vi "GdsLanguage_LoadLanguages.vi"(0 "LanguageFilesDirectory":path, 2 "LanguagesToLoad":T2, 3 "ChesumControl":T1, 5 "error in (no error)":errorcluster) -> (13 "StringIDsMissingThisLangaugeTranslation":string[](array[string]), 14 "StringIDArray":string[](array[string]), 16 "TranslatedStrings":string[](array[string]), 17 "DuplicateTranslations":string[](array[string]), 18 "FoundLanguages":T2[](array[typedef]), 19 "error out":errorcluster)   [LabVIEW 2020]
doc: "Load the languages (translated strings)."
uses:
  <resource>/Framework/Providers/Open_GDS/ClassProviders/Common/GdsLanguage/GdsLanguage_LanguageID.ctl
  <resource>/Framework/Providers/Open_GDS/ClassProviders/Common/GdsLanguage/private/GdsLanguage_ChecksumCheckType.ctl
  <resource>/Framework/Providers/Open_GDS/SubVIs/GOOP_ErrorCodes.ctl
  <vilib>/Utility/config.llb/Read Key (String).vi
  <vilib>/Utility/config.llb/NI_LVConfig.lvlib
panel:
  out "descriptions":string[](array[string])
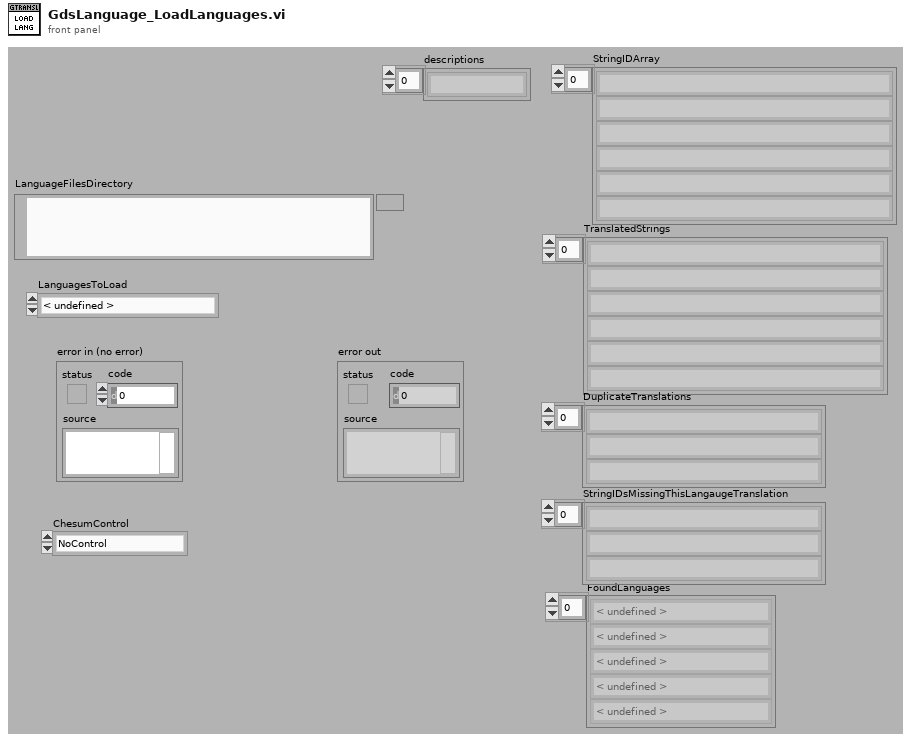
[diagram p1: front panel]
types:
  T1 = typedef "GdsLanguage_ChecksumCheckType.ctl" = enum16{"NoControl", "CheckChecksum", "AddChecksum"}
  T2 = typedef "GdsLanguage_LanguageID.ctl" = enum16{"< undefined >", "aa", "ab", "af", "am", "ar", "as", "ay", "az", "ba", "be", "bg", "bh", "bi", "bn", "bo", "br", "ca", "co", "cs", "cy", "da", "de", "dz", "el", "en", "eo", "es", "et", "eu", "fa", "fi", "fj", "fo", "fr", "fy", "ga", "gd", "gl", "gn", "gu", "gv", "ha", "he", "hi", "hr", "hu", "hy", "ia", "id", "ie", "ik", "is", "it", "iu", "ja", "jv", "ka", "kk", "kl", "km", "kn", "ko", "ks", "ku", "ky", "la", "li", "ln", "lo", "lt", "lv", "mg", "mi", "mk", "ml", "mn", "mo", "mr", "ms", "mt", "my", "na", "ne", "nl", "no", "oc", "om", "or", "pa", "pl", "ps", "pt", "qu", "rm", "rn", "ro", "ru", "rw", "sa", "sd", "sg", "sh", "si", "sk", "sl", "sm", "sn", "so", "sq", "sr", "ss", "st", "su", "sv", "sw", "ta", "te", "tg", "th", "ti", "tk", "tl", "tn", "to", "tr", "ts", "tt", "tw", "ug", "uk", "ur", "uz", "vi", "vo", "wo", "xh", "yi", "yo", "zh", "zu"}
  T3 = typedef "GOOP_ErrorCodes.ctl" = enum16{"LicenseFileMissing", "LicenseFileNotCorrect", "NoProductAccessGranted", "AgreementNoAccepted", "NoValidProviderFound", "LicenseExpired", "LanguageUndefined", "LanguageFileMissing", "LanguageFileChecksumError", "DublicateLanguageTranslation", "LanguageStringIDNotFound", "CommunityLimitReached", "ClassFileLocked", "ClassFileReadOnly", "ProjectNotValid"}
  T4 = typedef "NI_LVConfig.lvlib/Config Data RefNum.ctl" = refnum<k1>
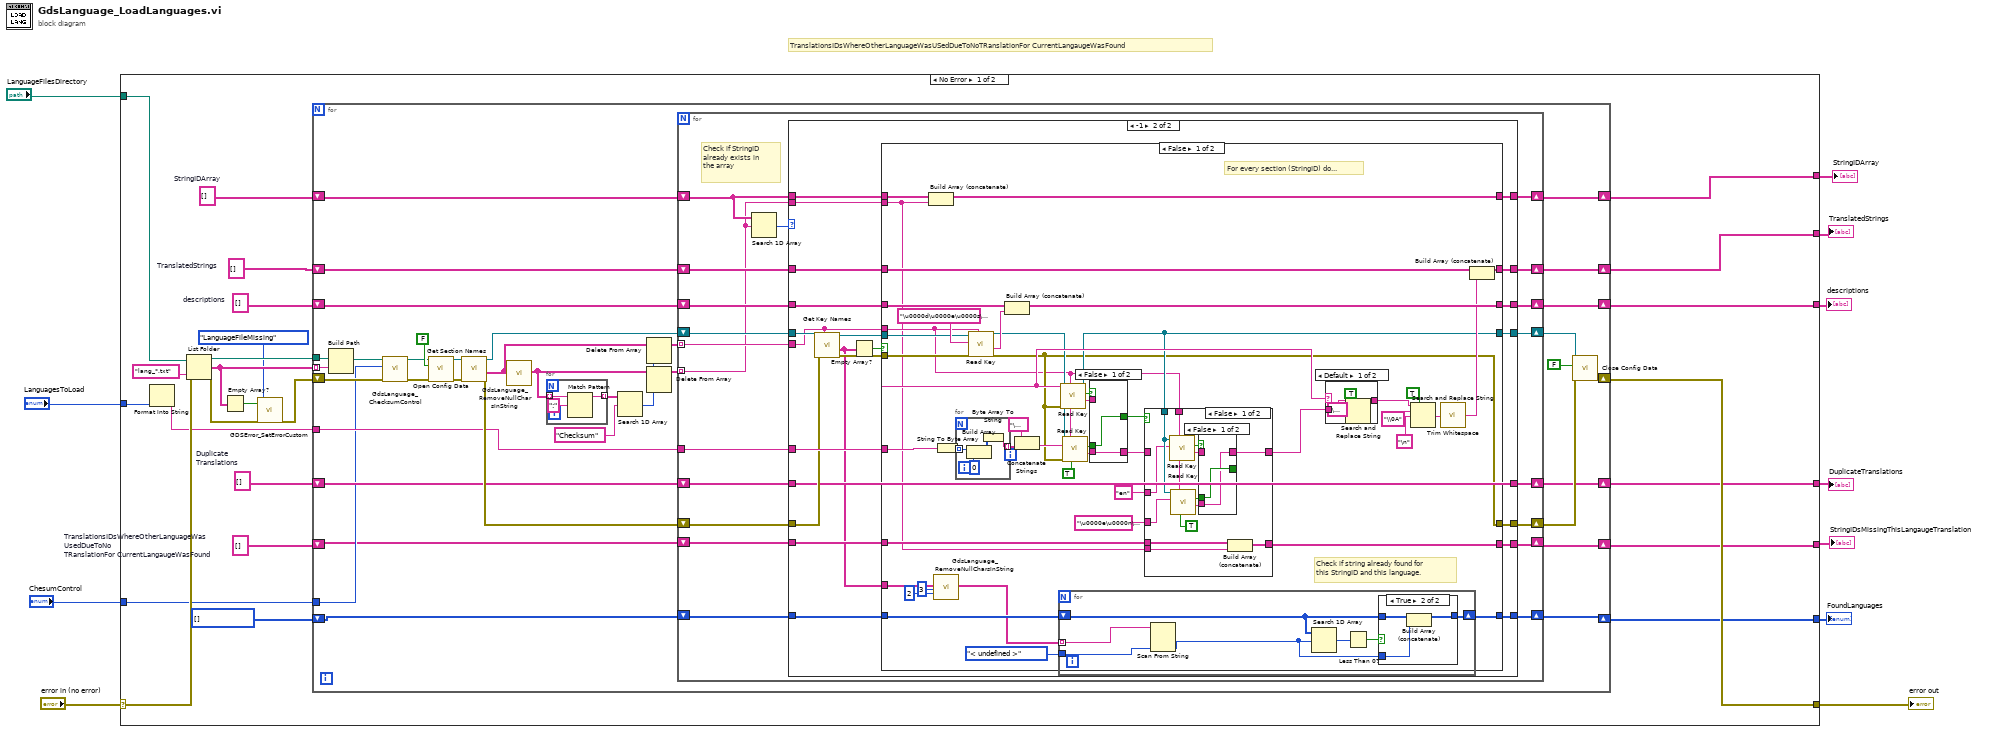
[diagram p0: block diagram]
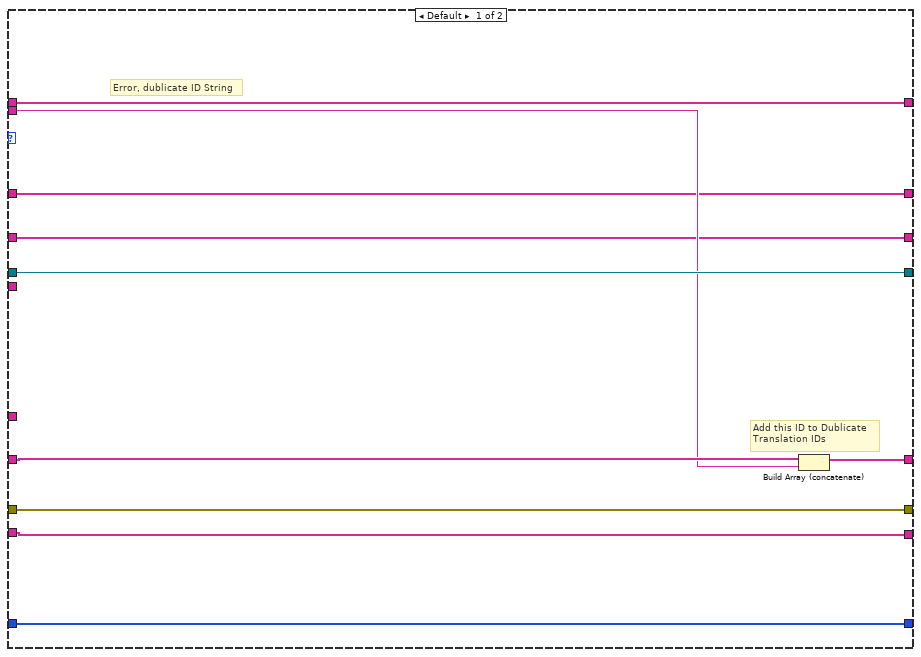
[diagram p2: hidden frame]
diagram:
  # "TranslationsIDsWhereOtherLanguageWasUSedDueToNoTRanslationFor CurrentLangaugeWasFound"
  n1 = case shown="No Error" "error in (no error)" {
    selector: "error in (no error)" -> [w32 w223]
    tunnel: [w33 w223] -> w10
    tunnel: "LanguageFilesDirectory" -> [w35 _]
    tunnel: "LanguagesToLoad" -> [w20 _]
    tunnel: [w29 _] -> w2
    tunnel: [w28 _] -> w7
    tunnel: [w26 _] -> w6
    tunnel: [w22 _] -> w5
    tunnel: [w23 _] -> w4
    tunnel: "ChesumControl" -> [w21 _]
    tunnel: [w17 _] -> w1
    frame No Error {
      w18 = string[] []  # TranslationsIDsWhereOtherLanguageWas UsedDueToNo TRanslationFor CurrentLangaugeWasFound
      w24 = string[] []  # descriptions
      w25 = T2[] [] items=["< undefined >", "aa", "ab", "af", "am", "ar", "as", "ay", "az", "ba", "be", "bg", "bh", "bi", "bn", "bo", "br", "ca", "co", "cs", "cy", "da", "de", "dz", "el", "en", "eo", "es", "et", "eu", "fa", "fi", "fj", "fo", "fr", "fy", "ga", "gd", "gl", "gn", "gu", "gv", "ha", "he", "hi", "hr", "hu", "hy", "ia", "id", "ie", "ik", "is", "it", "iu", "ja", "jv", "ka", "kk", "kl", "km", "kn", "ko", "ks", "ku", "ky", "la", "li", "ln", "lo", "lt", "lv", "mg", "mi", "mk", "ml", "mn", "mo", "mr", "ms", "mt", "my", "na", "ne", "nl", "no", "oc", "om", "or", "pa", "pl", "ps", "pt", "qu", "rm", "rn", "ro", "ru", "rw", "sa", "sd", "sg", "sh", "si", "sk", "sl", "sm", "sn", "so", "sq", "sr", "ss", "st", "su", "sv", "sw", "ta", "te", "tg", "th", "ti", "tk", "tl", "tn", "to", "tr", "ts", "tt", "tw", "ug", "uk", "ur", "uz", "vi", "vo", "wo", "xh", "yi", "yo", "zh", "zu"] ("Array out (String)")
      w27 = string[] []  # Duplicate Translations
      w30 = string[] []  # TranslatedStrings
      w31 = string[] []  # StringIDArray
      n2 = Format Into String(w20) -> (resulting string=w19:string)  [unwired: 3 in, 1 out]
      n3 = List Folder(path=w35, pattern="lang_*.txt", error in=w32) -> (path out=w34:path, filenames=w16:string[], error out=w13:errorcluster)  [unwired: 1 in, 1 out]
      n4 = Empty Array?(array=w16) -> (empty?=w14:bool)
      n5 = call <resource>:"GDSError_SetErrorCustom.vi"("status"=w14, "error in (no error)"=w13, "UserDefinedCodes(+5000)"=GOOP_ErrorCodes."LanguageFileMissing") -> ("error out"=w12:errorcluster)  [unwired: 16 in]
      n6 = for {
        tunnel: w34 -> [w65]
        tunnel: w16 -> [w64] mode=indexing
        tunnel: w19 -> [w63]
        shift-right: [w62] -> w33
        shift-left: w12 -> [w49]
        shift-right: [w59] -> w28
        shift-left: w31 -> [w61]
        shift-right: [w58] -> w29
        shift-left: w30 -> [w60]
        shift-right: [w56] -> w26
        shift-left: w27 -> [w57]
        shift-right: [w54] -> w22
        shift-left: w25 -> [w53]
        shift-right: [w51] -> w23
        shift-left: w24 -> [w52]
        tunnel: w21 -> [w46]
        shift-right: [w45] -> w17
        shift-left: w18 -> [w44]
        n7 = Build Path(base path=w65, name or relative path=w64) -> (appended path=w50:path)
        n8 = call <resource>:"GdsLanguage_ChecksumControl.vi"("error in"=w49, "ChesumControl"=w46, "LanguangeFileIn"=w50) -> ("error out"=w47:errorcluster, "LanguangeFileOut"=w48:path)  [unwired: 7 in]
        n9 = call <vilib>:"Open Config Data.vi"("error in (no error)"=w47, "create file if necessary (T)"=FALSE ("create file if necessary? (T)"), "configuration file path"=w48) -> ("error out"=w68:errorcluster, "refnum"=w72:T4)  [unwired: 6 in, 1 out]
        n10 = call <vilib>:"Get Section Names.vi"("error in (no error)"=w68, "refnum"=w72) -> ("error out"=w67:errorcluster, "section names"=w41:string[], "refnum out"=w70:T4)  [unwired: 7 in]
        n11 = call <resource>:"GdsLanguage_RemoveNullCharsInString.vi"("StringArray-IN"=w41) -> ("StringArray-Out"=w39:string[])  [unwired: 18 in]
        n12 = for {
          tunnel: w39 -> [w75] mode=indexing
          tunnel: [w73] -> w43 mode=indexing
          n13 = Match Pattern(string=w75, regular expression=":") -> (before substring=w73:string)  [unwired: 1 in, 3 out]
        }
        n14 = Search 1D Array(1D array=w43, element="Checksum") -> (index of element=w37:i32)  [unwired: 1 in]
        n15 = Delete From Array(array=w41, index=w37) -> (array with subset deleted=w40:string[])  [unwired: 1 in, 1 out]
        n16 = Delete From Array(array=w39, index=w37) -> (array with subset deleted=w38:string[])  [unwired: 1 in, 1 out]
        n17 = for {
          tunnel: w38 -> [w79] mode=indexing
          shift-right: [w95] -> w69
          shift-left: w70 -> [w87]
          tunnel: w63 -> [w94]
          shift-right: [w93] -> w66
          shift-left: w67 -> [w88]
          shift-right: [w78] -> w59
          shift-left: w61 -> [w80]
          shift-right: [w91] -> w58
          shift-left: w60 -> [w92]
          shift-right: [w89] -> w56
          shift-left: w57 -> [w90]
          shift-right: [w83] -> w54
          shift-left: w53 -> [w82]
          shift-right: [w85] -> w51
          shift-left: w52 -> [w86]
          tunnel: w40 -> [w84] mode=indexing
          shift-right: [w77] -> w45
          shift-left: w44 -> [w76]
          # "Check if StringID already exists in the array"
          n18 = Search 1D Array(1D array=w80, element=w79) -> (index of element=w81:i32)  [unwired: 1 in]
          n19 = case shown="-1" w81 {
            tunnel: [w102 w109] -> w95
            tunnel: w94 -> [_ w127]
            tunnel: [w103 w108] -> w93
            tunnel: w92 -> [w97 w126]
            tunnel: [w97 w125] -> w91
            tunnel: w90 -> [w104 w114]
            tunnel: [w105 w114] -> w89
            tunnel: w88 -> [w103 w124]
            tunnel: w87 -> [w102 w123]
            tunnel: w86 -> [w98 w122]
            tunnel: [w98 w119] -> w85
            tunnel: w84 -> [_ w110]
            tunnel: [w99 w118] -> w83
            tunnel: w82 -> [w99 w117]
            tunnel: w80 -> [w100 w116]
            tunnel: w79 -> [w101 w115]
            tunnel: [w100 w113] -> w78
            tunnel: [w96 w112] -> w77
            tunnel: w76 -> [w96 w111]
            frame Default {
              # "Add this ID to Dublicate\nTranslation IDs"
              # "Error, dublicate ID String"
              n20 = Build Array (concatenate)(w104, w101) -> (w105:string[])
            }
            frame -1 {
              n21 = call <vilib>:"Get Key Names.vi"("section"=w110, "error in (no error)"=w124, "refnum"=w123) -> ("error out"=w120:errorcluster, "key names"=w107:string[], "refnum out"=w121:T4)  [unwired: 5 in, 1 out]
              n22 = Empty Array?(array=w107) -> (empty?=w106:bool)
              n23 = case shown="False" w106 {
                tunnel: w127 -> [w172 _]
                tunnel: w126 -> [w171 w221]
                tunnel: [w170 w221] -> w125
                tunnel: w122 -> [w167 w220]
                tunnel: w121 -> [w166 w219]
                tunnel: w120 -> [w164 w218]
                tunnel: [w163 w220] -> w119
                tunnel: [w160 w216] -> w118
                tunnel: w117 -> [w159 w216]
                tunnel: w116 -> [w148 w222]
                tunnel: w115 -> [w130 _]
                tunnel: [w147 w222] -> w113
                tunnel: [w139 w217] -> w112
                tunnel: w111 -> [w138 w217]
                tunnel: w110 -> [w131 _]
                tunnel: [w137 w219] -> w109
                tunnel: [w134 w218] -> w108
                tunnel: w107 -> [w133 _]
                frame False {
                  # "Check if string already found for \nthis StringID and this language."
                  # "For every section (StringID) do..."
                  n24 = Build Array (concatenate)(w148, w130) -> (w147:string[])
                  n25 = call <resource>:"GdsLanguage_RemoveNullCharsInString.vi"("StringArray-IN"=w133, "MaxLengthLimit(ignored if not wired)"=3, "MinLengthLimit(ignored if not wired)"=2) -> ("StringArray-Out"=w132:string[])  [unwired: 16 in]
                  n26 = String To Byte Array(string=w172) -> (unsigned byte array=w151:u8[])
                  n27 = for {
                    tunnel: w151 -> [w204] mode=indexing
                    tunnel: [w202] -> w157 mode=indexing
                    n28 = Build Array(w204, u8 0 ("element")) -> (w203:u8[])
                    n29 = Byte Array To String(unsigned byte array=w203) -> (string=w202:string)
                  }
                  n30 = call-poly <vilib>:"Read Key.vi"("section"=w131, "error in (no error)"=w164, "key"="\u0000d\u0000e\u0000s\u0000c\u0000r\u0000i\u0000p\u0000t\u0000i\u0000o\u0000n\u0000", "refnum"=w166) -> ("error out"=w134:errorcluster, "value"=w168:string, "refnum out"=w165:T4)  [unwired: 4 in, 1 out]
                  n31 = Build Array (concatenate)(w167, w168) -> (w163:string[])
                  n32 = Concatenate Strings("\u0000" ("string"), w157) -> (w154:string)
                  n33 = for {
                    shift-right: [w209] -> w160
                    shift-left: w159 -> [w210]
                    tunnel: w132 -> [w207] mode=indexing
                    tunnel: GdsLanguage_LanguageID."< undefined >" ("LanguagesToLoad") -> [w206]
                    n34 = Scan From String(input string=w207, default 1=w206) -> (output 1=w205:T2)  [unwired: 3 in, 3 out]
                    n35 = Search 1D Array(1D array=w210, element=w205) -> (index of element=w208:i32)  [unwired: 1 in]
                    n36 = Less Than 0?(x=w208) -> (x < 0?=w211:bool)
                    n37 = case shown="True" w211 {
                      tunnel: w205 -> [_ w215]
                      tunnel: w210 -> [w212 w214]
                      tunnel: [w212 w213] -> w209
                      frame False {
                      }
                      frame True {
                        n38 = Build Array (concatenate)(w214, w215) -> (w213:T2[])
                      }
                    }
                  }
                  n39 = call-poly <vilib>:"Read Key.vi"("section"=w131, "error in (no error)"=w134, "key"=w172, "refnum"=w165) -> ("value"=w155:string, "found?"=w156:bool, "refnum out"=w137:T4)  [unwired: 4 in, 1 out]
                  n40 = call-poly <vilib>:"Read Key.vi"("read raw string? (F)"=TRUE, "section"=w131, "error in (no error)"=w134, "key"=w154, "refnum"=w165) -> ("value"=w152:string, "found?"=w153:bool)  [unwired: 3 in, 2 out]
                  n41 = case shown="False" w156 {
                    selector: w156 -> [_ w200]
                    tunnel: [w198 w200] -> w140
                    tunnel: w155 -> [_ w199]
                    tunnel: [w197 w199] -> w136
                    tunnel: w153 -> [w198 _]
                    tunnel: w152 -> [w197 _]
                    frame False {
                    }
                    frame True {
                    }
                  }
                  n42 = case shown="False" w140 {
                    tunnel: [w185 w191] -> w139
                    tunnel: w138 -> [w184 w191]
                    tunnel: w131 -> [w176 _]
                    tunnel: "\u0000e\u0000n\u0000" ("string") -> [w178 _]
                    tunnel: w137 -> [w177 _]
                    tunnel: w136 -> [_ w190]
                    tunnel: [w175 w190] -> w135
                    tunnel: w130 -> [w174 _]
                    tunnel: "en" ("string") -> [w173 _]
                    frame False {
                      n43 = call-poly <vilib>:"Read Key.vi"("section"=w176, "key"=w173, "refnum"=w177) -> ("value"=w180:string, "found?"=w179:bool)  [unwired: 5 in, 2 out]
                      n44 = call-poly <vilib>:"Read Key.vi"("read raw string? (F)"=TRUE, "section"=w176, "key"=w178, "refnum"=w177) -> ("value"=w182:string, "found?"=w181:bool)  [unwired: 4 in, 2 out]
                      n45 = case shown="False" w179 {
                        selector: w179 -> [_ w189]
                        tunnel: [w187 w189] -> _
                        tunnel: w180 -> [_ w188]
                        tunnel: [w186 w188] -> w175
                        tunnel: w181 -> [w187 _]
                        tunnel: w182 -> [w186 _]
                        frame False {
                        }
                        frame True {
                        }
                      }
                      n46 = Build Array (concatenate)(w184, w174) -> (w185:string[])
                    }
                    frame True {
                    }
                  }
                  n47 = case shown="Default" w172 {
                    tunnel: [w193 w196] -> w146
                    tunnel: w135 -> [w192 w196]
                    frame Default {
                      n48 = Search and Replace String(replace all?=TRUE ("replace all? (F)"), input string=w192, search string="\u0000" ("string")) -> (result string=w193:string)  [unwired: 5 in, 3 out]
                    }
                    frame "zh" {
                    }
                  }
                  n49 = Search and Replace String(replace all?=TRUE ("replace all? (F)"), input string=w146, search string="\\0A", replace string="\n" ("search string")) -> (result string=w142:string)  [unwired: 4 in, 3 out]
                  n50 = call <vilib>:"Trim Whitespace.vi"("string"=w142) -> ("trimmed string"=w141:string)  [unwired: 1 in]
                  n51 = Build Array (concatenate)(w171, w141) -> (w170:string[])
                }
                frame True {
                }
              }
            }
          }
        }
        n52 = call <vilib>:"Close Config Data.vi"("error in (no error)"=w66, "write file if changed (T)"=FALSE ("write configuration file? (T)"), "refnum"=w69) -> ("error out"=w62:errorcluster)  [unwired: 7 in, 1 out]
      }
    }
    frame Error {
    }
  }
  "error out" <- w10
  "TranslatedStrings" <- w2
  "StringIDArray" <- w7
  "DuplicateTranslations" <- w6
  "FoundLanguages" <- w5
  "descriptions" <- w4
  "StringIDsMissingThisLangaugeTranslation" <- w1
